vi "SLL DE Virtual Graph.vi"(8 "error in(no error)":errorcluster) -> (0 "error Out":errorcluster)   [LabVIEW 2009]
uses:
  Controls/SLL DE Get Plot LV2Global Parameters.ctl
  Sub VIs/DAQ Engine/Controls/SLL DE List of Analog Inputs.ctl
  Controls/SLL DE Virtual Graph Options.ctl
  Sub VIs/DAQ Engine/Controls/SLL DE DAQ Global Options.ctl
  Sub VIs/DAQ Engine/Controls/SLL DE DAQ Global Elements.ctl
  Controls/SLL DE Get Plot LV2Global Options.ctl
  Sub VIs/DAQ Engine/Controls/SLL DE Circular Buffer Pointers List.ctl
  Sub VIs/DAQ Engine/Controls/SLL DE Circular Buffer Options.ctl
  <vilib>/Utility/miscctls.llb/LVAnnotationListTypeDef.ctl
  Controls/SLL DE Virtual Chart Datalog Driver Options.ctl
  Sub VIs/DAQ Engine/Controls/SLL DE DO Command LV2Global Options.ctl
  Controls/SLL DE File Logging Command List.ctl
panel:
  out "Time :":string="12:11:16 PM"
  out "Date :":string="08-25-2009"
  in  "Enable Record":bool caption="Record All channels"
  in  "Plot 4":u16(ring)=19 caption="Y-Axis(1)" items=["FM01TS", "FM02TS", "FM03TS", "FM04TS", "FM05TS", "PC01TS", "PC02TS", "PC03TS", "PT01TS", "PT02TS", "PT03TS", "PT04TS", "PT05TS", "PT06TS", "ST01TS", "TC01TS", "TC02TS", "TC03TS", "TT01TS", "None"]
  in  "Plot 3":u16(ring)=19 caption="Y-Axis(1)" items=["FM01TS", "FM02TS", "FM03TS", "FM04TS", "FM05TS", "PC01TS", "PC02TS", "PC03TS", "PT01TS", "PT02TS", "PT03TS", "PT04TS", "PT05TS", "PT06TS", "ST01TS", "TC01TS", "TC02TS", "TC03TS", "TT01TS", "None"]
  in  "Plot 2":u16(ring)=19 caption="Y-Axis(1)" items=["FM01TS", "FM02TS", "FM03TS", "FM04TS", "FM05TS", "PC01TS", "PC02TS", "PC03TS", "PT01TS", "PT02TS", "PT03TS", "PT04TS", "PT05TS", "PT06TS", "ST01TS", "TC01TS", "TC02TS", "TC03TS", "TT01TS", "None"]
  in  "Y-Axis 2":bool=TRUE
  in  "Y-Axis 1":bool=TRUE
  in  "Plot 1":u16(ring) caption="Y-Axis(1)" items=["FM01TS", "FM02TS", "FM03TS", "FM04TS", "FM05TS", "PC01TS", "PC02TS", "PC03TS", "PT01TS", "PT02TS", "PT03TS", "PT04TS", "PT05TS", "PT06TS", "ST01TS", "TC01TS", "TC02TS", "TC03TS", "TT01TS", "None"]
  in  "Hold Update":bool=TRUE
  in  "X-Scale":u16(ring)=19 caption="Y-Axis(1)" items=["FM01TS", "FM02TS", "FM03TS", "FM04TS", "FM05TS", "PC01TS", "PC02TS", "PC03TS", "PT01TS", "PT02TS", "PT03TS", "PT04TS", "PT05TS", "PT06TS", "ST01TS", "TC01TS", "TC02TS", "TC03TS", "TT01TS", "Time Scale"]
  out "Graph":T1(graph)
  in  "List of Analog Inputs":T2
  in  "Data Cluster":T4={"Record"=FALSE, "Datalog Folder Path"=path "D:/Projects/Projects/Eaton Prop Valve Test Stand/Software/Info/Datalog File Path/Back up.dat", "Graph - Interval b/w Samples"=0, "AI Sampling Rate (Samples/Sec)"=3.0, "Data Log To csv File"=[], "File - Interval b/w Samples"=0, "Time Array"=[], "Graph Mod"=0, "File Mod"=0, "Plot Details"={"Sample Value In"=[], "Plot 1"=FALSE, "Plot 2"=FALSE, "Plot 3"=FALSE, "Plot 4"=FALSE}}
  in  "Data Save Folder Path":path=path "D:/STI Projects/DAQ Engine/SLL DAQ Engine/Software/Info/Report"
  in  "Snap Shot":bool caption="Duplicate SupFile"
  in  "Restart Plot":bool
  in  "Exit":bool
  in  "Print":bool
  # "Logo"
  # "Logo"
  # "<Project Name>"
  # "Graphical Display"
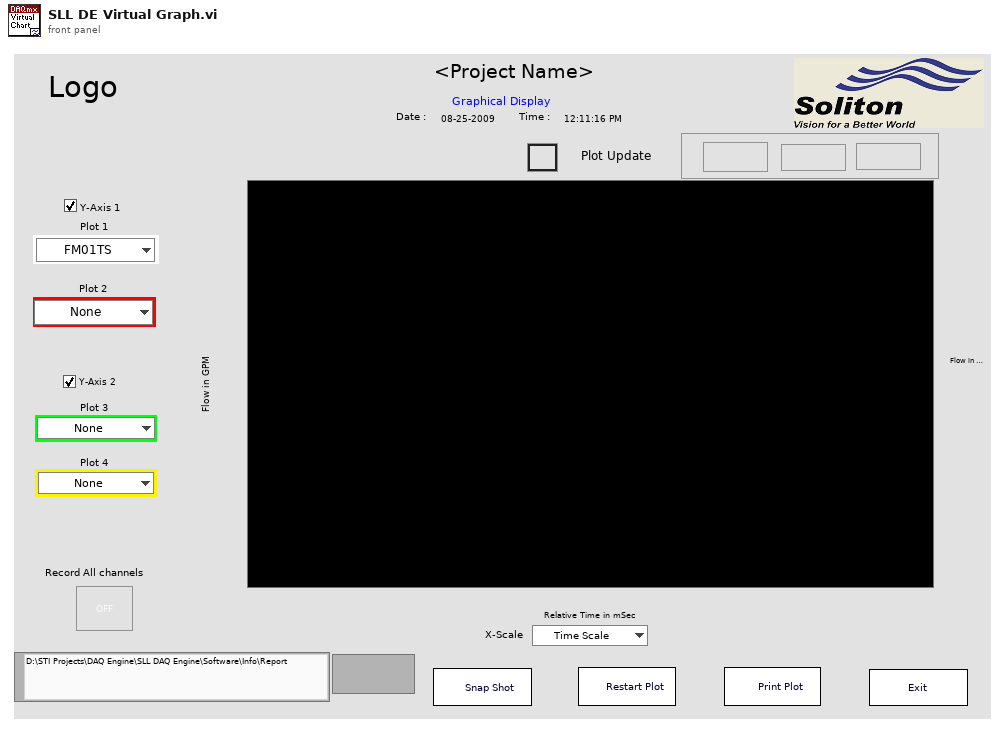
[diagram p1: front panel]
types:
  T1 = cluster{"Sample Value In":sgl[], "Sample Value In":sgl[]}[]
  T2 = typedef "SLL DE List of Analog Inputs.ctl" = enum16{"None"}
  T3 = typedef "SLL DE Get Plot LV2Global Parameters.ctl" = cluster{"Sample Value In":sgl[][], "Plot 1":bool, "Plot 2":bool, "Plot 3":bool, "Plot 4":bool}
  T4 = cluster{"Record":bool, "Datalog Folder Path":path, "Graph - Interval b/w Samples":i32, "AI Sampling Rate (Samples/Sec)":dbl, "Data Log To csv File":sgl[][], "File - Interval b/w Samples":i32, "Time Array":timestamp[], "Graph Mod":i32, "File Mod":i32, "Plot Details":T3}
  T5 = typedef "SLL DE Virtual Graph Options.ctl" = enum16{"Initialize", "Initialize Channel List", "Check Channel Type", "Update Graph Parameters", "Poll Events", "Get Values", "Config Plot", "Plot Ramp", "Datalog", "Add Plot Name", "Enable Record", "Snap Shot", "Restart", "Print Plot", "Error", "Exit"}
  T6 = typedef "SLL DE DAQ Global Options.ctl" = enum16{"Init", "Write 1", "Read 1", "Write Array", "Read Array", "Clear"}
  T7 = typedef "SLL DE DAQ Global Elements.ctl" = enum16{"AI Error", "AO Error", "DI Error", "DO Error", "AI Restart", "DI Restart", "AI Running", "AO Running", "DI Running", "DO Running", "DAQ Exit?"}
  T8 = typedef "SLL DE Get Plot LV2Global Options.ctl" = enum16{"Init", "Get Plot", "Read Plot"}
  T9 = typedef "SLL DE Circular Buffer Pointers List.ctl" = enum16{"Graph Pointer", "File Log Pointer", "Pointer 3", "Pointer 4"}
  T10 = typedef "SLL DE Circular Buffer Options.ctl" = enum16{"Initialize", "Init Pointer X", "Write", "Read Single Value", "Read Pointer X (Multi Value)", "Clear Data"}
  T11 = typedef "LVAnnotationListTypeDef.ctl" = cluster{"Name":string, "Color":u32, "Style":u8, "Point Style":u8, "Name Visible":bool, "Allow Drag":bool, "Annotation Mode":u32, "Plot":i32, "Index":i32, "Position":cluster{"X":dbl, "Y":dbl}, "X Scale":u32, "Y Scale":u32, "Show Arrow":bool, "Lock Name":bool, "Plot Area":i32, "Label Offset":cluster{"X":dbl, "Y":dbl}}[]
  T12 = typedef "SLL DE Virtual Chart Datalog Driver Options.ctl" = enum16{"Initialise", "Write Headings", "Write", "Check File Size", "Read", "Clear"}
  T13 = typedef "SLL DE File Logging Command List.ctl" = enum16{"Start Logging", "Stop Logging"}
  T14 = typedef "SLL DE DO Command LV2Global Options.ctl" = enum16{"Init/Register Events", "Get Event Refnum", "Fire Event", "Distroy Event"}
  T15 = cluster{"Plot 1":string, "Plot 2":string, "Plot 3":string, "Plot 4":string, "X Scale":string, "Y-Axis 2":bool, "Y-Axis 1":bool}
  T16 = typedef "SLL DE List of AI Channel Type.ctl" = enum16{"Pressure", "Flow", "Temperature", "Time Scale", "Voltage", "Current", "Frequency", "Sound", "Speed", "Torque", "Distance", "Channel Type 1", "Channel Type 2", "Channel Type 3"}
  T17 = cluster{"Time Scale":sgl[], "Sample Value In":sgl[]}[]
  T18 = enum16{"Left Button", "Center Button", "Right Button", "Window Close"}
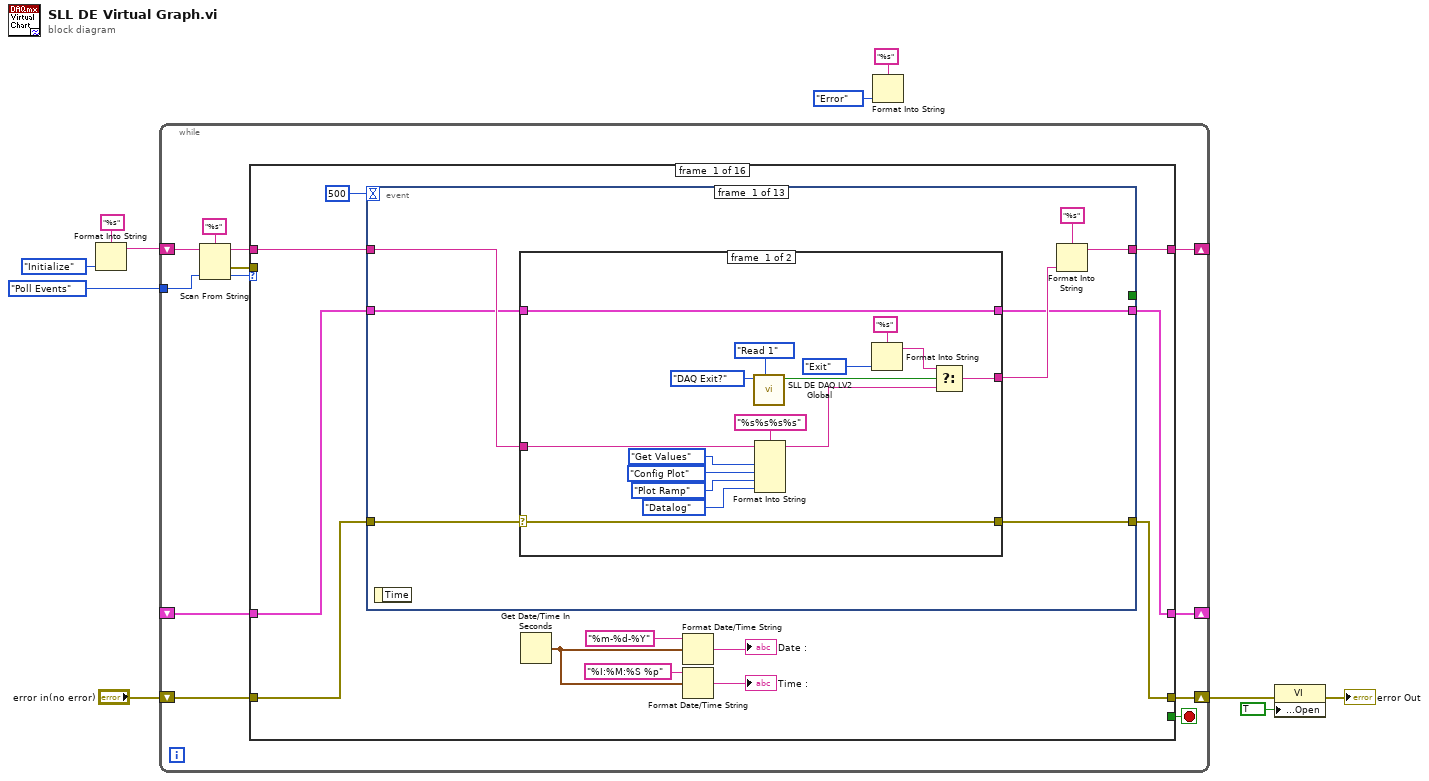
[diagram p0: block diagram]
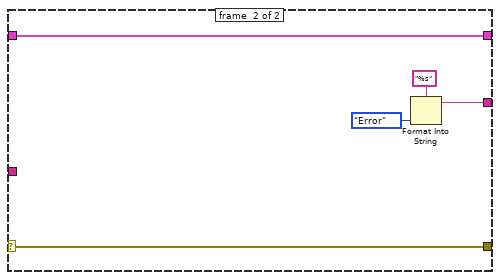
[diagram p2: hidden frame]
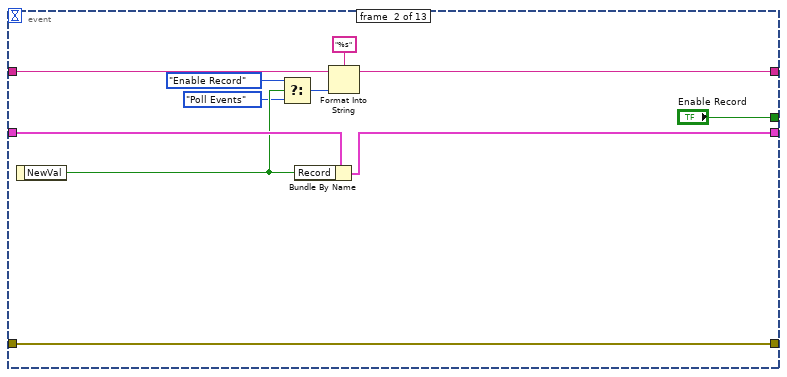
[diagram p3: hidden frame]
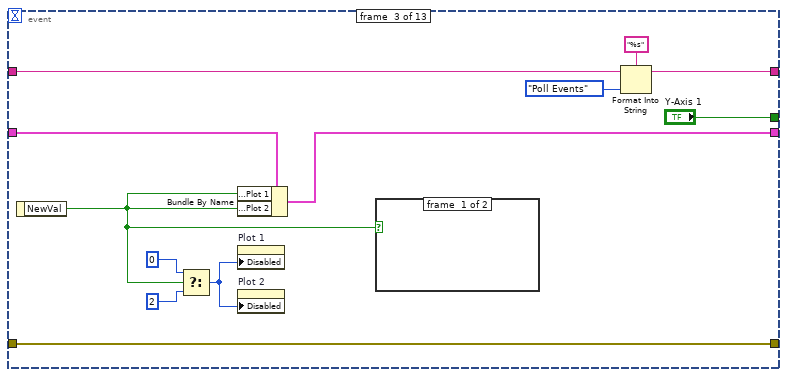
[diagram p4: hidden frame]
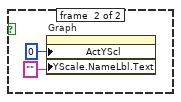
[diagram p5: hidden frame]
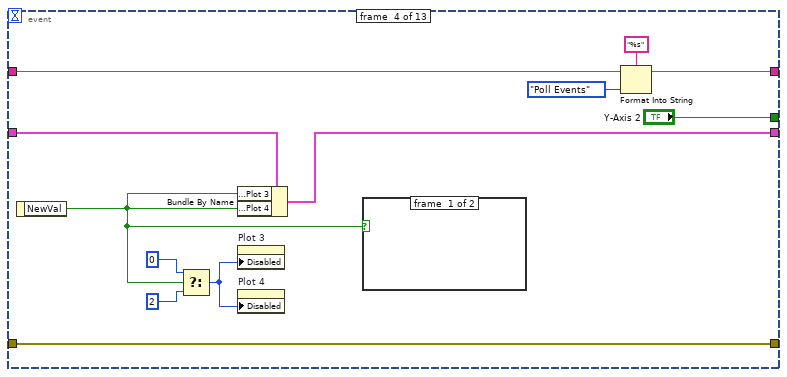
[diagram p6: hidden frame]
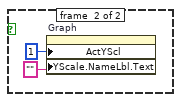
[diagram p7: hidden frame]
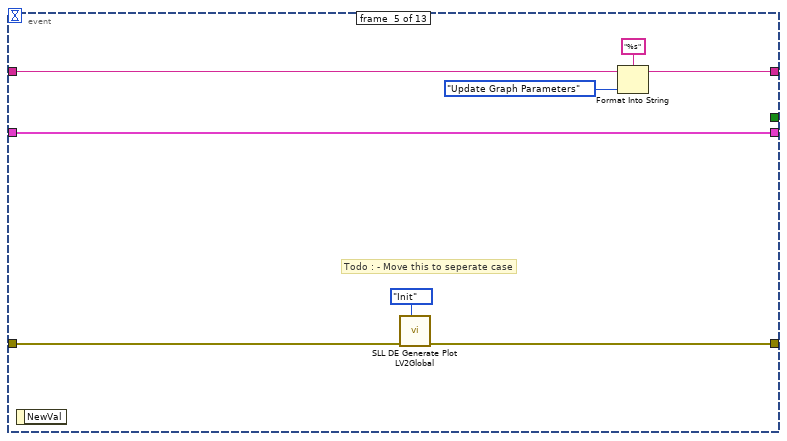
[diagram p8: hidden frame]
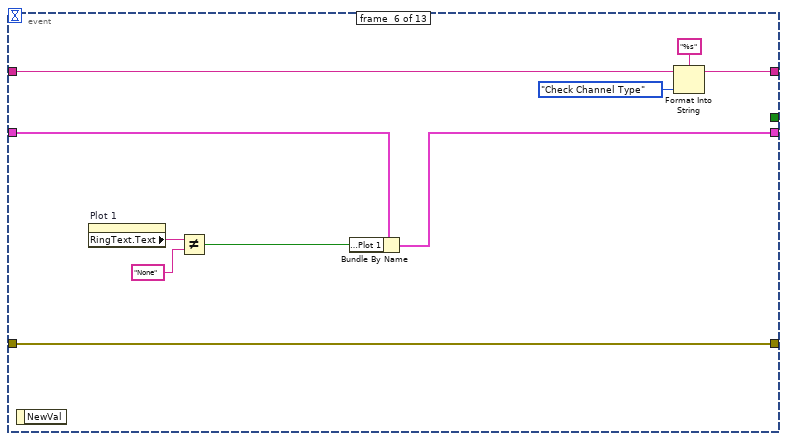
[diagram p9: hidden frame]
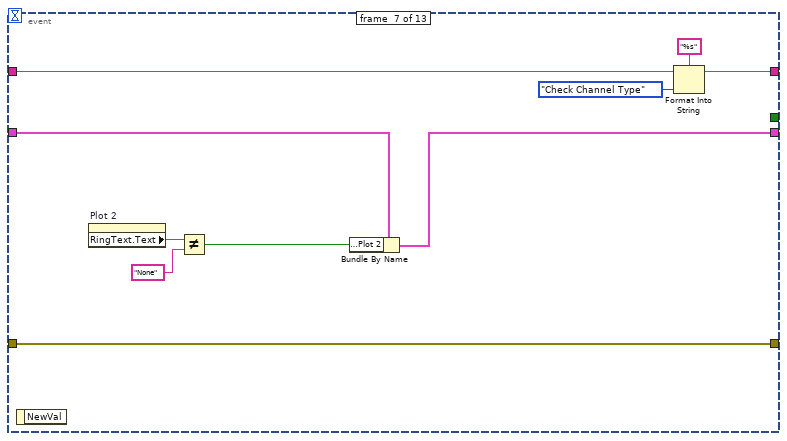
[diagram p10: hidden frame]
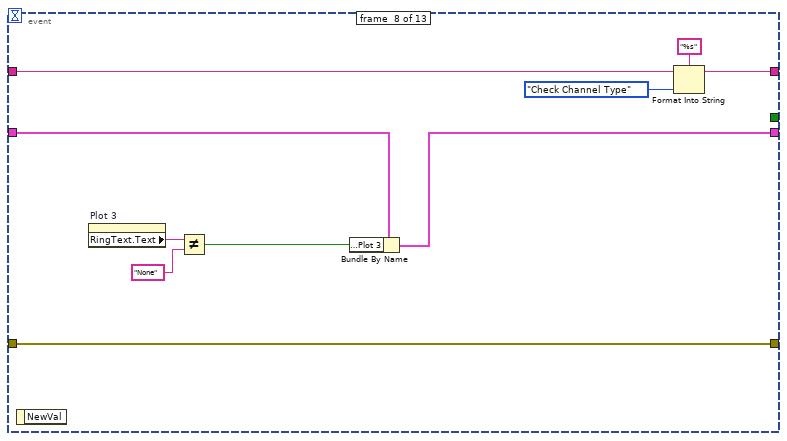
[diagram p11: hidden frame]
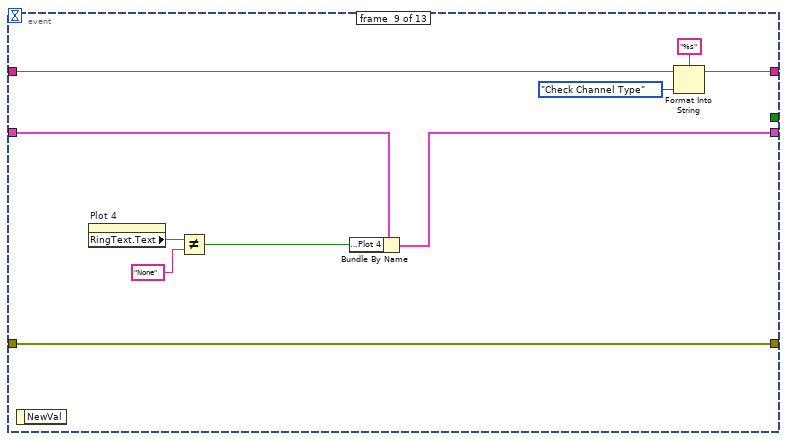
[diagram p12: hidden frame]
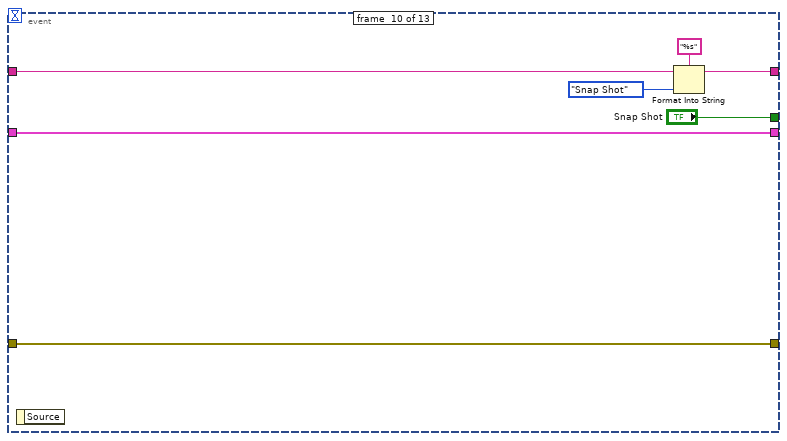
[diagram p13: hidden frame]
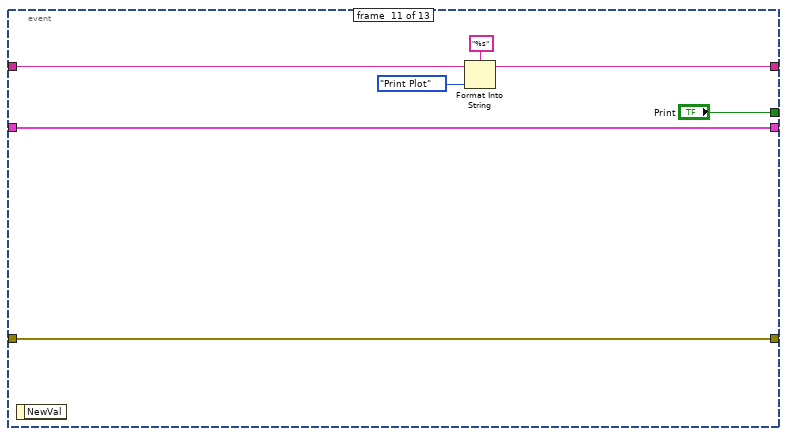
[diagram p14: hidden frame]
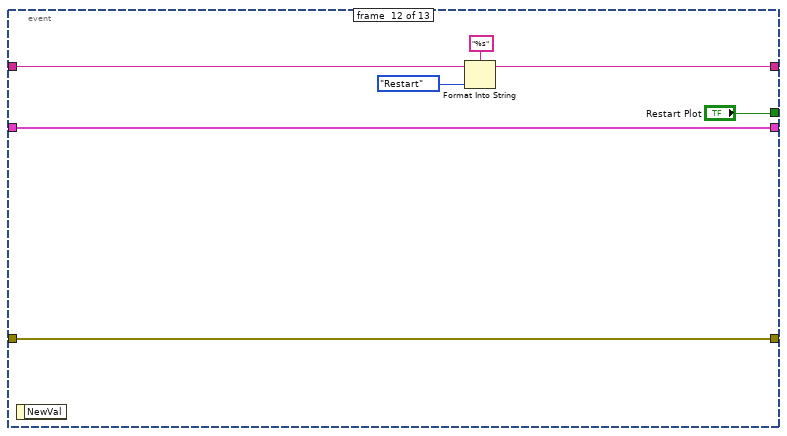
[diagram p15: hidden frame]
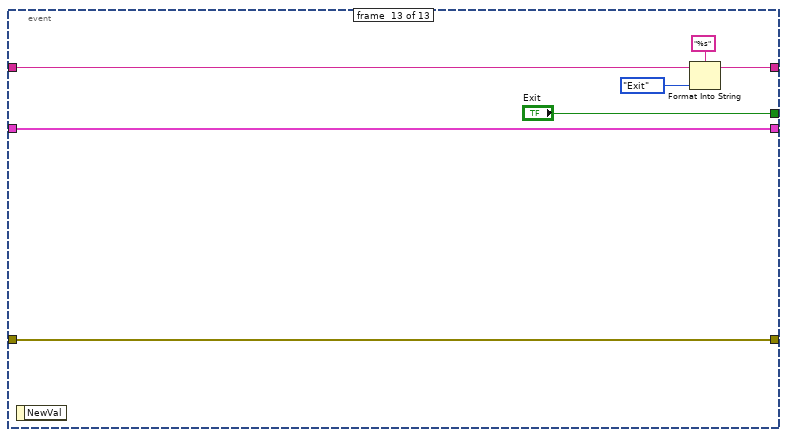
[diagram p16: hidden frame]
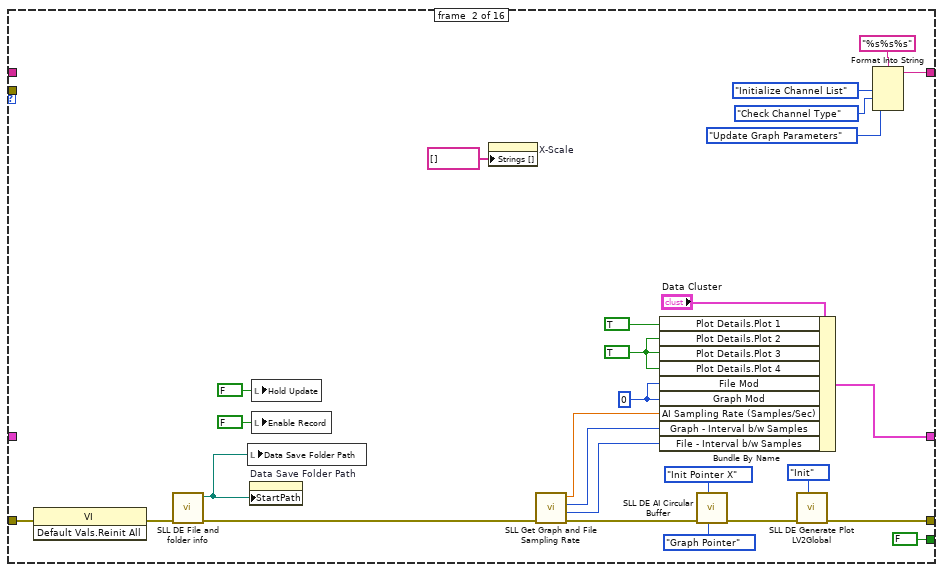
[diagram p17: hidden frame]
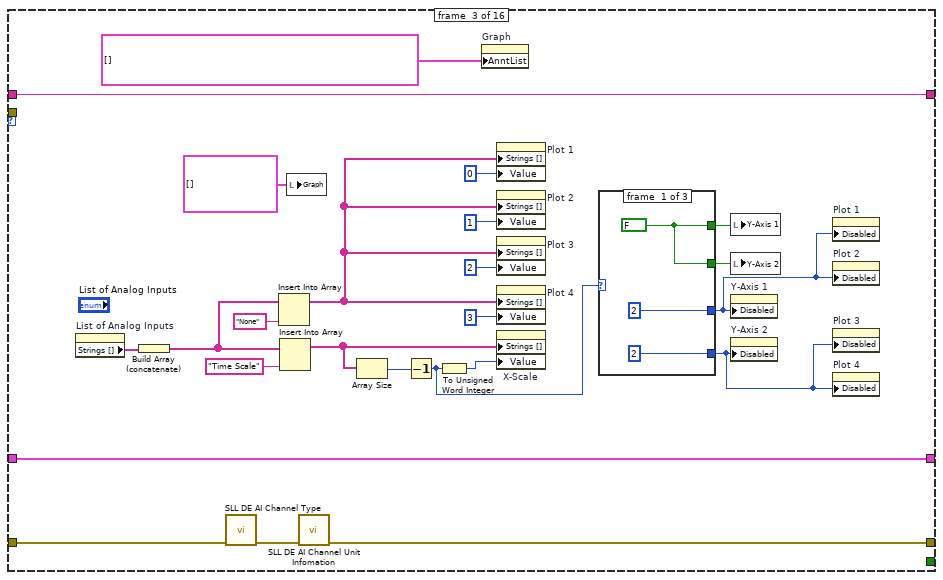
[diagram p18: hidden frame]
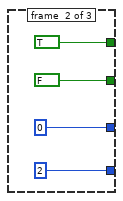
[diagram p19: hidden frame]
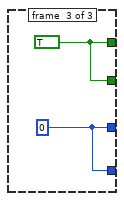
[diagram p20: hidden frame]
diagram:
  n1 = Format Into String(format string="%s", SLL_DE_Virtual_Graph_Options."Initialize" ("SLL DE Virtual Chart Options")) -> (resulting string=w10:string)  [unwired: 2 in, 1 out]
  n2 = while {
    shift-right: [w19] -> _
    shift-left: w10 -> [w22]
    shift-right: [w18] -> _
    shift-left: _ -> [w16]
    shift-right: [w15] -> w8
    shift-left: "error in(no error)" -> [w14]
    tunnel: SLL_DE_Virtual_Graph_Options."Poll Events" ("SLL DE Virtual Chart Options") -> [w12]
    stop <- w17 stop-if-true
    n3 = Scan From String(format string="%s", input string=w22, default 1=w12) -> (remaining string=w20:string, error out=w13:errorcluster, output 1=w21:T5)  [unwired: 2 in, 1 out]
    n4 = case shown="\"Initialize\"" w21 {
      tunnel: w20 -> [w33 _ w217 w257 _ w349 w379 w391 w414 w428 w450 w464 _ w495 _ w513]
      tunnel: [w32 w198 w217 w256 w292 w349 w379 w391 w414 w428 w450 w464 w465 w495 w497 w513] -> w19
      tunnel: [w30 w202 w216 w249 w300 w350 w380 w387 w413 w425 w449 w461 w478 w484 w498 w512] -> w18
      tunnel: [_ FALSE _ _ _ _ _ _ _ _ _ _ FALSE _ _ TRUE] -> w17
      tunnel: w16 -> [w31 _ w216 w250 w300 w344 w381 w387 w413 w425 w449 w461 w478 w484 w498 w512]
      tunnel: [w28 w192 w209 w261 w299 w345 w375 w386 w418 w426 w440 w451 w474 w480 w496 w508] -> w15
      tunnel: w14 -> [w29 w205 w211 w261 w301 w346 w378 w390 w419 w427 w434 w454 w475 w485 w500 w509]
      tunnel: w13 -> [_ _ _ _ _ _ _ _ _ _ _ _ _ _ _ _]
      frame #0 {
        n5 = event shown="[5] \"Plot 1\": Value Change" {
          selector: _ -> [_ _ _ _ _ _ _ _ _ _ _ _ _]
          dyn-events: _ -> [_ _ _ _ _ _ _ _ _ _ _ _ _]
          timeout: 500 -> [_ _ _ _ _ _ _ _ _ _ _ _ _]
          tunnel: w33 -> [w39 w64 w81 w91 w107 w111 w121 w131 w141 w153 w158 w166 w172]
          tunnel: [w41 w73 w82 w92 w109 w119 w122 w132 w142 w154 w162 w170 w177] -> w32
          tunnel: [_ "Enable Record" "Y-Axis 1" "Y-Axis 2" _ _ _ _ _ "Snap Shot" "Print" "Restart Plot" "Exit"] -> _
          tunnel: w31 -> [w37 w71 w85 w90 w103 w118 w125 w135 w145 w152 w161 w169 w175]
          tunnel: [w36 w70 w84 w93 w103 w117 w123 w133 w143 w152 w161 w169 w175] -> w30
          tunnel: w29 -> [w38 w69 w79 w94 w105 w116 w124 w134 w144 w155 w160 w168 w174]
          tunnel: [w35 w69 w79 w94 w104 w116 w124 w134 w144 w155 w160 w168 w174] -> w28
          event #0 {
            n6 = event-data() -> ()  [unwired: 1 in, 1 out]
            n7 = case shown="No Error" w38 {
              selector: w38 -> [w43 w59]
              tunnel: [w58 w61] -> w40
              tunnel: w39 -> [w45 _]
              tunnel: w37 -> [w44 w60]
              tunnel: [w44 w60] -> w36
              tunnel: [w43 w59] -> w35
              frame #0 {
                n8 = call "SLL DE DAQ LV2 Global.vi"("Option"=SLL_DE_DAQ_Global_Options."Read 1", "Element"=SLL_DE_DAQ_Global_Elements."DAQ Exit?") -> ("Status Out"=w55:bool)  [unwired: 7 in, 2 out]
                n9 = Format Into String(format string="%s%s%s%s", initial string=w45, SLL_DE_Virtual_Graph_Options."Get Values" ("SLL DE Virtual Chart Options"), SLL_DE_Virtual_Graph_Options."Config Plot" ("SLL DE Virtual Chart Options"), SLL_DE_Virtual_Graph_Options."Plot Ramp" ("SLL DE Virtual Chart Options"), SLL_DE_Virtual_Graph_Options."Datalog" ("SLL DE Virtual Chart Options")) -> (resulting string=w49:string)  [unwired: 1 in, 1 out]
                n10 = Format Into String(format string="%s", SLL_DE_Virtual_Graph_Options."Exit" ("SLL DE Virtual Chart Options")) -> (resulting string=w46:string)  [unwired: 2 in, 1 out]
                n11 = Select(t=w46, s=w55, f=w49) -> (s? t:f=w58:string)
              }
              frame #1 {
                n12 = Format Into String(format string="%s", SLL_DE_Virtual_Graph_Options."Error" ("SLL DE Virtual Chart Options")) -> (resulting string=w61:string)  [unwired: 2 in, 1 out]
              }
            }
            n13 = Format Into String(format string="%s", w40) -> (resulting string=w41:string)  [unwired: 2 in, 1 out]
          }
          event #1 {
            n14 = event-data() -> ("NewVal"=w67:bool)  [unwired: 1 in]
            n15 = Select(t=SLL_DE_Virtual_Graph_Options."Enable Record" ("SLL DE Virtual Chart Options"), s=w67, f=SLL_DE_Virtual_Graph_Options."Poll Events") -> (s? t:f=w66:T5)
            n16 = Bundle By Name(cluster=w71, "Record"=w67) -> (w70:T4)
            n17 = Format Into String(format string="%s", initial string=w64, w66) -> (resulting string=w73:string)  [unwired: 1 in, 1 out]
          }
          event #2 {
            n18 = event-data() -> ("NewVal"=w75:bool)  [unwired: 1 in]
            n19 = Select(t=u8 0 ("Disabled"), s=w75, f=u8 2 ("Disabled")) -> (s? t:f=w77:u8)
            n20 = Bundle By Name(cluster=w85, "Plot Details.Plot 1"=w75, "Plot Details.Plot 2"=w75) -> (w84:T4)
            n21 = property on="Plot 1" class="Ring (strict)"("Disabled"=w77) -> ()  [unwired: 2 in, 2 out]
            n22 = property on="Plot 2" class="Ring (strict)"("Disabled"=w77) -> ()  [unwired: 2 in, 2 out]
            n23 = case shown="True" w75 {
              frame #0 {
              }
              frame #1 {
                n24 = property on="Graph" class="XYGraph (strict)"("ActYScl"=0 ("Active Y Scale"), "YScale.NameLbl.Text"="" ("Y Scale.Name Label.Text")) -> ()  [unwired: 2 in, 2 out]
              }
            }
            n25 = Format Into String(format string="%s", initial string=w81, SLL_DE_Virtual_Graph_Options."Poll Events" ("SLL DE Virtual Chart Options")) -> (resulting string=w82:string)  [unwired: 1 in, 1 out]
          }
          event #3 {
            n26 = event-data() -> ("NewVal"=w89:bool)  [unwired: 1 in]
            n27 = Select(t=u8 0 ("Disabled"), s=w89, f=u8 2 ("Disabled")) -> (s? t:f=w96:u8)
            n28 = Bundle By Name(cluster=w90, "Plot Details.Plot 3"=w89, "Plot Details.Plot 4"=w89) -> (w93:T4)
            n29 = property on="Plot 3" class="Ring (strict)"("Disabled"=w96) -> ()  [unwired: 2 in, 2 out]
            n30 = property on="Plot 4" class="Ring (strict)"("Disabled"=w96) -> ()  [unwired: 2 in, 2 out]
            n31 = case shown="True" w89 {
              frame #0 {
              }
              frame #1 {
                n32 = property on="Graph" class="XYGraph (strict)"("ActYScl"=1 ("Active Y Scale"), "YScale.NameLbl.Text"="" ("Y Scale.Name Label.Text")) -> ()  [unwired: 2 in, 2 out]
              }
            }
            n33 = Format Into String(format string="%s", initial string=w91, SLL_DE_Virtual_Graph_Options."Poll Events" ("SLL DE Virtual Chart Options")) -> (resulting string=w92:string)  [unwired: 1 in, 1 out]
          }
          event #4 {
            # "Todo : - Move this to seperate case"
            n34 = event-data() -> ()  [unwired: 1 in, 1 out]
            n35 = call "SLL DE Generate Plot LV2Global.vi"("Option"=SLL_DE_Get_Plot_LV2Global_Options."Init", "error in (no error)"=w105) -> ("error IO"=w104:errorcluster)  [unwired: 8 in, 1 out]
            n36 = Format Into String(format string="%s", initial string=w107, SLL_DE_Virtual_Graph_Options."Update Graph Parameters" ("SLL DE Virtual Chart Options")) -> (resulting string=w109:string)  [unwired: 1 in, 1 out]
          }
          event #5 {
            n37 = event-data() -> ()  [unwired: 1 in, 1 out]
            n38 = property on="Plot 1" class="Ring (strict)"() -> ("RingText.Text"=w115:string)  [unwired: 2 in, 2 out]
            n39 = Not Equal?(x=w115, y="None") -> (x != y?=w113:bool)
            n40 = Bundle By Name(cluster=w118, "Plot Details.Plot 1"=w113) -> (w117:T4)
            n41 = Format Into String(format string="%s", initial string=w111, SLL_DE_Virtual_Graph_Options."Check Channel Type" ("SLL DE Virtual Chart Options")) -> (resulting string=w119:string)  [unwired: 1 in, 1 out]
          }
          event #6 {
            n42 = event-data() -> ()  [unwired: 1 in, 1 out]
            n43 = property on="Plot 2" class="Ring (strict)"() -> ("RingText.Text"=w129:string)  [unwired: 2 in, 2 out]
            n44 = Not Equal?(x=w129, y="None") -> (x != y?=w127:bool)
            n45 = Bundle By Name(cluster=w125, "Plot Details.Plot 2"=w127) -> (w123:T4)
            n46 = Format Into String(format string="%s", initial string=w121, SLL_DE_Virtual_Graph_Options."Check Channel Type" ("SLL DE Virtual Chart Options")) -> (resulting string=w122:string)  [unwired: 1 in, 1 out]
          }
          event #7 {
            n47 = event-data() -> ()  [unwired: 1 in, 1 out]
            n48 = property on="Plot 3" class="Ring (strict)"() -> ("RingText.Text"=w139:string)  [unwired: 2 in, 2 out]
            n49 = Not Equal?(x=w139, y="None") -> (x != y?=w137:bool)
            n50 = Bundle By Name(cluster=w135, "Plot Details.Plot 3"=w137) -> (w133:T4)
            n51 = Format Into String(format string="%s", initial string=w131, SLL_DE_Virtual_Graph_Options."Check Channel Type" ("SLL DE Virtual Chart Options")) -> (resulting string=w132:string)  [unwired: 1 in, 1 out]
          }
          event #8 {
            n52 = event-data() -> ()  [unwired: 1 in, 1 out]
            n53 = property on="Plot 4" class="Ring (strict)"() -> ("RingText.Text"=w149:string)  [unwired: 2 in, 2 out]
            n54 = Not Equal?(x=w149, y="None") -> (x != y?=w147:bool)
            n55 = Bundle By Name(cluster=w145, "Plot Details.Plot 4"=w147) -> (w143:T4)
            n56 = Format Into String(format string="%s", initial string=w141, SLL_DE_Virtual_Graph_Options."Check Channel Type" ("SLL DE Virtual Chart Options")) -> (resulting string=w142:string)  [unwired: 1 in, 1 out]
          }
          event #9 {
            n57 = event-data() -> ()  [unwired: 1 in, 1 out]
            n58 = Format Into String(format string="%s", initial string=w153, SLL_DE_Virtual_Graph_Options."Snap Shot" ("SLL DE Virtual Chart Options")) -> (resulting string=w154:string)  [unwired: 1 in, 1 out]
          }
          event #10 {
            n59 = event-data() -> ()  [unwired: 1 in, 1 out]
            n60 = Format Into String(format string="%s", initial string=w158, SLL_DE_Virtual_Graph_Options."Print Plot" ("SLL DE Virtual Chart Options")) -> (resulting string=w162:string)  [unwired: 1 in, 1 out]
          }
          event #11 {
            n61 = event-data() -> ()  [unwired: 1 in, 1 out]
            n62 = Format Into String(format string="%s", initial string=w166, SLL_DE_Virtual_Graph_Options."Restart" ("SLL DE Virtual Chart Options")) -> (resulting string=w170:string)  [unwired: 1 in, 1 out]
          }
          event #12 {
            n63 = event-data() -> ()  [unwired: 1 in, 1 out]
            n64 = Format Into String(format string="%s", initial string=w172, SLL_DE_Virtual_Graph_Options."Exit" ("SLL DE Virtual Chart Options")) -> (resulting string=w177:string)  [unwired: 1 in, 1 out]
          }
        }
        n65 = Get Date/Time In Seconds() -> (seconds since 1Jan1904=w25:timestamp)
        n66 = Format Date/Time String(time format string (%c)="%m-%d-%Y", seconds (now)=w25) -> (date/time string=→"Date :":string)  [unwired: 1 in]
        n67 = Format Date/Time String(time format string (%c)="%I:%M:%S %p", seconds (now)=w25) -> (date/time string=→"Time :":string)  [unwired: 1 in]
      }
      frame #1 {
        w190 = TRUE ("Data Cluster 2.Plot 1")
        w195 = 0 ("Mod")
        n68 = invoke class="VI" method="Default Vals.Reinit All"(error in=w205) -> (error out=w204:errorcluster)  [unwired: 2 in, 2 out]
        n69 = call "SLL DE File and folder info.vi"("error in (no error)"=w204) -> ("error out"=w187:errorcluster, "Report path"=w181:path)  [unwired: 5 in, 4 out]
        n70 = local write "Data Save Folder Path"(w181) -> ()
        n71 = property on="Data Save Folder Path" class="Path"("StartPath"=w181) -> ()  [unwired: 2 in, 2 out]
        n72 = local write "Hold Update"(FALSE ("Hold Update")) -> ()
        n73 = local write "Enable Record"(FALSE ("Enable Record")) -> ()
        n74 = property on="X-Scale" class="Ring (strict)"("Strings []"=string[] []) -> ()  [unwired: 2 in, 2 out]
        n75 = call "SLL Get Graph and File Sampling Rate.vi"("error in (no error)"=w187) -> ("error out"=w186:errorcluster, "File - Interval b/w Samples"=w184:i32, "Graph - Interval b/w Samples"=w179:i32, "AI Sampling Rate (Samples/Sec)"=w185:dbl)  [unwired: 7 in]
        n76 = Bundle By Name(cluster="Data Cluster", "Plot Details.Plot 1"=TRUE ("Data Cluster 2.Plot 1"), "Plot Details.Plot 2"=w190, "Plot Details.Plot 3"=w190, "Plot Details.Plot 4"=w190, "File Mod"=w195, "Graph Mod"=w195, "AI Sampling Rate (Samples/Sec)"=w185, "Graph - Interval b/w Samples"=w179, "File - Interval b/w Samples"=w184) -> (w202:T4)
        n77 = call "SLL DE AI Circular Buffer.vi"("Pointers"=SLL_DE_Circular_Buffer_Pointers_List."Graph Pointer", "Options"=SLL_DE_Circular_Buffer_Options."Init Pointer X" ("AI Option"), "error in (no error)"=w186) -> ("error Out"=w193:errorcluster)  [unwired: 3 in, 5 out]
        n78 = call "SLL DE Generate Plot LV2Global.vi"("Option"=SLL_DE_Get_Plot_LV2Global_Options."Init", "error in (no error)"=w193) -> ("error IO"=w192:errorcluster)  [unwired: 8 in, 1 out]
        n79 = Format Into String(format string="%s%s%s", SLL_DE_Virtual_Graph_Options."Initialize Channel List" ("SLL DE Virtual Chart Options"), SLL_DE_Virtual_Graph_Options."Check Channel Type" ("SLL DE Virtual Chart Options"), SLL_DE_Virtual_Graph_Options."Update Graph Parameters" ("SLL DE Virtual Chart Options")) -> (resulting string=w198:string)  [unwired: 2 in, 1 out]
      }
      frame #2 {
        n80 = property on="List of Analog Inputs" class="Enum (strict)"() -> ("Strings []"=w221:string[])  [unwired: 2 in, 2 out]
        n81 = Build Array (concatenate)(w221) -> (w220:string[])
        n82 = call "SLL DE AI Channel Type.vi"("error in (no error)"=w211) -> ("error out"=w210:errorcluster)  [unwired: 7 in, 3 out]
        n83 = Insert Into Array(array=w220, new element="None") -> (w222:string[])  [unwired: 1 in]
        n84 = Insert Into Array(array=w220, new element="Time Scale") -> (w223:string[])  [unwired: 1 in]
        n85 = local write "Graph"(T1 [] ("Graph")) -> ()
        n86 = call "SLL DE AI Channel Unit Infomation.vi"("error in (no error)"=w210) -> ("error out"=w209:errorcluster)  [unwired: 9 in, 1 out]
        n87 = Array Size(array=w223) -> (size(s)=w224:i32)
        n88 = Decrement(x=w224) -> (x-1=w226:i32)
        n89 = To Unsigned Word Integer(number=w226) -> (unsigned 16bit integer=w225:u16)
        n90 = property on="Graph" class="XYGraph (strict)"("AnntList"=T11 [] ("Annotation List")) -> ()  [unwired: 2 in, 2 out]
        n91 = property on="Plot 1" class="Ring (strict)"("Strings []"=w222, "Value"=u16 0) -> ()  [unwired: 2 in, 2 out]
        n92 = property on="Plot 2" class="Ring (strict)"("Strings []"=w222, "Value"=u16 1) -> ()  [unwired: 2 in, 2 out]
        n93 = property on="Plot 3" class="Ring (strict)"("Strings []"=w222, "Value"=u16 2) -> ()  [unwired: 2 in, 2 out]
        n94 = property on="Plot 4" class="Ring (strict)"("Strings []"=w222, "Value"=u16 3) -> ()  [unwired: 2 in, 2 out]
        n95 = property on="X-Scale" class="Ring (strict)"("Strings []"=w223, "Value"=w225) -> ()  [unwired: 2 in, 2 out]
        n96 = case shown="0" w226 {
          tunnel: [w232 TRUE w238] -> w227
          tunnel: [w232 FALSE w238] -> w228
          tunnel: [u8 2 ("Disabled") u8 0 ("Disabled") w237] -> w208
          tunnel: [u8 2 ("Disabled") u8 2 ("Disabled") w237] -> w207
          frame #0 {
            w232 = FALSE
          }
          frame #1 {
          }
          frame #2 {
            w237 = u8 0 ("Disabled")
            w238 = TRUE
          }
        }
        n97 = local write "Y-Axis 1"(w227) -> ()
        n98 = local write "Y-Axis 2"(w228) -> ()
        n99 = property on="Y-Axis 1" class="Bool (strict)"("Disabled"=w208) -> ()  [unwired: 2 in, 2 out]
        n100 = property on="Y-Axis 2" class="Bool (strict)"("Disabled"=w207) -> ()  [unwired: 2 in, 2 out]
        n101 = property on="Plot 1" class="Ring (strict)"("Disabled"=w208) -> ()  [unwired: 2 in, 2 out]
        n102 = property on="Plot 2" class="Ring (strict)"("Disabled"=w208) -> ()  [unwired: 2 in, 2 out]
        n103 = property on="Plot 3" class="Ring (strict)"("Disabled"=w207) -> ()  [unwired: 2 in, 2 out]
        n104 = property on="Plot 4" class="Ring (strict)"("Disabled"=w207) -> ()  [unwired: 2 in, 2 out]
      }
      frame #3 {
        n105 = Unbundle By Name(w250) -> ("Plot Details.Plot 2"=w252:bool, "Plot Details.Plot 4"=w251:bool)
        n106 = property on="Plot 3" class="Ring (strict)"() -> ("RingText.Text"=w254:string)  [unwired: 2 in, 2 out]
        n107 = property on="Plot 4" class="Ring (strict)"() -> ("RingText.Text"=w253:string)  [unwired: 2 in, 2 out]
        n108 = property on="Plot 1" class="Ring (strict)"() -> ("RingText.Text"=w255:string)  [unwired: 2 in, 2 out]
        n109 = property on="Plot 2" class="Ring (strict)"() -> ("RingText.Text"=w260:string)  [unwired: 2 in, 2 out]
        n110 = case shown="Default" w254 {
          selector: w254 -> [_ w267]
          tunnel: w253 -> [_ w271]
          tunnel: [FALSE TRUE] -> w242
          tunnel: [w262 w265] -> w241
          tunnel: w251 -> [w262 w264]
          frame #0 {
          }
          frame #1 {
            n111 = call "SLL DE Virtual Graph Channel Parameters.vi"("Virtual Channel Name"=w267) -> ("Channel Type"=w270:T16)  [unwired: 5 in, 5 out]
            n112 = call "SLL DE Virtual Graph Channel Parameters.vi"("Virtual Channel Name"=w271) -> ("Channel Type"=w269:T16)  [unwired: 5 in, 5 out]
            n113 = Not Equal?(x=w270, y=w269) -> (x != y?=w268:bool)
            n114 = case shown="True" w268 {
              tunnel: [w272 FALSE] -> w265
              tunnel: w264 -> [w272 _]
              frame #0 {
              }
              frame #1 {
                n115 = property on="Plot 2" class="Ring (strict)"() -> ("NumItems"=w274:u32)  [unwired: 2 in, 2 out]
                n116 = Decrement(x=w274) -> (x-1=w273:u32)
                n117 = local write "Plot 4"(w273) -> ()
              }
            }
          }
        }
        n118 = case shown="Default" w255 {
          selector: w255 -> [_ w281]
          tunnel: w260 -> [_ w285]
          tunnel: [FALSE TRUE] -> w247
          tunnel: [w276 w279] -> w246
          tunnel: w252 -> [w276 w278]
          frame #0 {
          }
          frame #1 {
            n119 = call "SLL DE Virtual Graph Channel Parameters.vi"("Virtual Channel Name"=w281) -> ("Channel Type"=w284:T16)  [unwired: 5 in, 5 out]
            n120 = call "SLL DE Virtual Graph Channel Parameters.vi"("Virtual Channel Name"=w285) -> ("Channel Type"=w283:T16)  [unwired: 5 in, 5 out]
            n121 = Not Equal?(x=w284, y=w283) -> (x != y?=w282:bool)
            n122 = case shown="True" w282 {
              tunnel: [w286 FALSE] -> w279
              tunnel: w278 -> [w286 _]
              frame #0 {
              }
              frame #1 {
                n123 = property on="Plot 2" class="Ring (strict)"() -> ("NumItems"=w288:u32)  [unwired: 2 in, 2 out]
                n124 = Decrement(x=w288) -> (x-1=w287:u32)
                n125 = local write "Plot 2"(w287) -> ()
              }
            }
          }
        }
        n126 = local read "Y-Axis 1"() -> (w245:bool)
        n127 = local read "Y-Axis 2"() -> (w240:bool)
        n128 = And(x=w245, y=w247) -> (x .and. y?=w248:bool)
        n129 = And(x=w245, y=w246) -> (x .and. y?=w244:bool)
        n130 = And(x=w242, y=w240) -> (x .and. y?=w243:bool)
        n131 = And(x=w240, y=w241) -> (x .and. y?=w239:bool)
        n132 = Bundle By Name(cluster=w250, "Plot Details.Plot 1"=w248, "Plot Details.Plot 2"=w244, "Plot Details.Plot 3"=w243, "Plot Details.Plot 4"=w239) -> (w249:T4)
        n133 = Format Into String(format string="%s", initial string=w257, SLL_DE_Virtual_Graph_Options."Update Graph Parameters" ("SLL DE Virtual Chart Options")) -> (resulting string=w256:string)  [unwired: 1 in, 1 out]
      }
      frame #4 {
        n134 = property on="X-Scale" class="Ring (strict)"(error in=w301) -> (error out=w298:errorcluster, "RingText.Text"=w291:string)  [unwired: 1 in, 1 out]
        n135 = property on="Plot 1" class="Ring (strict)"(error in=w301) -> (error out=w302:errorcluster, "RingText.Text"=w303:string)  [unwired: 1 in, 1 out]
        n136 = property on="Plot 3" class="Ring (strict)"(error in=w301) -> ("RingText.Text"=w304:string)  [unwired: 1 in, 2 out]
        n137 = Build Array(w303, w304) -> (w305:string[])
        n138 = case shown="Default" w291 {
          selector: w291 -> [_ w308]
          tunnel: w298 -> [w307 w310]
          frame #0 {
            n139 = property on="Graph" class="XYGraph (strict)"(error in=w307, "XScale.NameLbl.Text"="Relative Time in mSec" ("X Scale.Name Label.Text")) -> ()  [unwired: 1 in, 2 out]
          }
          frame #1 {
            n140 = call "SLL DE Virtual Graph Channel Parameters.vi"("error in (no error)"=w310, "Virtual Channel Name"=w308) -> ("error out"=w309:errorcluster, "Maximum Value"=w312:dbl, "Minimum Value"=w313:dbl, "Graph Name Label"=w314:string, "Increment"=w311:dbl)  [unwired: 4 in, 1 out]
            n141 = property on="Graph" class="XYGraph (strict)"(error in=w309, "XScale.NameLbl.Text"=w314, "XScale.Minimum"=w313, "XScale.Maximum"=w312, "XScale.Increment"=w311) -> ()  [unwired: 1 in, 2 out]
          }
        }
        n142 = for {
          tunnel: w305 -> [w319] mode=indexing
          shift-right: [w318] -> w299
          shift-left: w302 -> [w317]
          i -> [w320]
          n143 = property on="Graph" class="XYGraph (strict)"(error in=w317, "ActYScl"=w320) -> (error out=w316:errorcluster)  [unwired: 1 in, 1 out]
          n144 = call "SLL DE Virtual Graph Channel Parameters.vi"("error in (no error)"=w316, "Virtual Channel Name"=w319) -> ("error out"=w315:errorcluster, "Maximum Value"=w323:dbl, "Minimum Value"=w322:dbl, "Graph Name Label"=w321:string, "Increment"=w324:dbl)  [unwired: 4 in, 1 out]
          n145 = property on="Graph" class="XYGraph (strict)"(error in=w315, "YScale.NameLbl.Text"=w321, "YScale.Minimum"=w322, "YScale.Maximum"=w323, "YScale.Increment"=w324) -> (error out=w318:errorcluster)  [unwired: 1 in, 1 out]
        }
        n146 = Format Into String(format string="%s%s%s%s%s", SLL_DE_Virtual_Graph_Options."Get Values" ("SLL DE Virtual Chart Options"), SLL_DE_Virtual_Graph_Options."Config Plot" ("SLL DE Virtual Chart Options"), SLL_DE_Virtual_Graph_Options."Plot Ramp" ("SLL DE Virtual Chart Options"), SLL_DE_Virtual_Graph_Options."Datalog" ("SLL DE Virtual Chart Options"), SLL_DE_Virtual_Graph_Options."Add Plot Name" ("SLL DE Virtual Chart Options")) -> (resulting string=w292:string)  [unwired: 2 in, 1 out]
      }
      frame #5 {
        n147 = call "SLL DE AI Circular Buffer.vi"("Pointers"=SLL_DE_Circular_Buffer_Pointers_List."Graph Pointer", "Options"=SLL_DE_Circular_Buffer_Options."Read Pointer X (Multi Value)" ("AI Option"), "error in (no error)"=w346) -> ("error Out"=w345:errorcluster, "Output Data"=w343:sgl[][], "Multi Time Stamp"=w330:timestamp[])  [unwired: 3 in, 3 out]
        n148 = Unbundle By Name(w344) -> ("Graph Mod"=w337:i32, "Graph - Interval b/w Samples"=w340:i32, "Record"=w336:bool, "File Mod"=w335:i32, "File - Interval b/w Samples"=w333:i32)
        n149 = Transpose 2D Array(2D array=w343) -> (transposed array=w329:sgl[][])
        n150 = Array Size(array=w329) -> (size(s)=w342:i32[])
        n151 = Index Array(array=w342) -> (element #1=w331:i32, element #2=w332:i32)  [unwired: 2 in]
        n152 = case shown="True" w336 {
          tunnel: w333 -> [_ w358]
          tunnel: w329 -> [_ w365]
          tunnel: w332 -> [_ w361]
          tunnel: w335 -> [w352 w357]
          tunnel: [sgl[][] [] ("Data Array Out") w360] -> w327
          tunnel: [w352 w359] -> w334
          tunnel: w331 -> [_ w356]
          tunnel: w330 -> [_ w355]
          tunnel: [timestamp[] [] ("Multi Time Stamp") w354] -> w328
          frame #0 {
          }
          frame #1 {
            n153 = Quotient & Remainder(x=w361, y=w358) -> (floor(x/y)=w364:i32)  [unwired: 1 out]
            n154 = Initialize Array(sgl 0.0, w356, w364) -> (w363:sgl[][])
            n155 = call "SLL DE Decimate 2D Array.vi"("Multi Time Stamp"=w355, "Ref Array"=w363, "Decimation Rate"=w358, "Mod"=w357, "Data Array"=w365) -> ("Time array"=w354:timestamp[], "Mod Out"=w359:i32, "Data Array Out"=w360:sgl[][])  [unwired: 3 in, 1 out]
          }
        }
        n156 = Quotient & Remainder(x=w332, y=w340) -> (floor(x/y)=w325:i32)  [unwired: 1 out]
        n157 = Initialize Array(sgl 0.0, w331, w325) -> (w339:sgl[][])
        n158 = call "SLL DE Decimate 2D Array.vi"("Multi Time Stamp"=w330, "Ref Array"=w339, "Decimation Rate"=w340, "Mod"=w337, "Data Array"=w329) -> ("Mod Out"=w338:i32, "Data Array Out"=w326:sgl[][])  [unwired: 3 in, 2 out]
        n159 = Bundle By Name(cluster=w344, "Plot Details.Sample Value In"=w326, "Graph Mod"=w338, "Data Log To csv File"=w327, "File Mod"=w334, "Time Array"=w328) -> (w350:T4)
      }
      frame #6 {
        # "This case wil execute when Enable Record button is clicked.\nAll the Pre- Recording conditions are performed in this case after which \nrecording is done in \"Continue Recording\" Case. eg. opening the datalog\nfile and stuffs."
        n160 = Get Date/Time In Seconds() -> (seconds since 1Jan1904=w369:timestamp)
        n161 = Format Date/Time String(time format string (%c)="%m_%Y_%d_%H_%M_%S", seconds (now)=w369) -> (date/time string=w373:string)  [unwired: 1 in]
        n162 = Concatenate Strings("Log_" ("string"), w373, ".csv" ("string")) -> (w368:string)
        n163 = Build Path(base path="Data Save Folder Path", name or relative path=w368) -> (appended path=w366:path)
        n164 = Bundle By Name(cluster=w381, "Datalog Folder Path"=w366) -> (w380:T4)
        n165 = disable-structure shown="Disabled" {
          frame #0 {
            n166 = call "SLL DE File Looging Command LV2Global.vi"("Option"=SLL_DE_DO_Command_LV2Global_Options."Fire Event", "File Logging Option"=SLL_DE_File_Logging_Command_List."Start Logging") -> ()  [unwired: 1 in, 9 out]
          }
          frame #1 {
          }
        }
        n167 = call "SLL DE csv File Driver.vi"("Datalog Driver Cases"=SLL_DE_Virtual_Chart_Datalog_Driver_Options."Initialise", "error in(no error)"=w378, "Datalog path (use dialog)"=w366) -> ("error out"=w376:errorcluster)  [unwired: 4 in, 4 out]
        n168 = call "SLL DE csv File Driver.vi"("Datalog Driver Cases"=SLL_DE_Virtual_Chart_Datalog_Driver_Options."Write Headings", "error in(no error)"=w376) -> ("error out"=w375:errorcluster)  [unwired: 5 in, 4 out]
      }
      frame #7 {
        n169 = Unbundle By Name(w387) -> ("Time Array"=w384:timestamp[], "Data Log To csv File"=w385:sgl[][], "Record"=w388:bool, "Datalog Folder Path"=w389:path)
        n170 = case shown="True" w388 {
          tunnel: w390 -> [w392 w403]
          tunnel: [w392 w398] -> w386
          tunnel: w389 -> [_ w401]
          tunnel: w385 -> [_ w397]
          tunnel: w384 -> [_ w396]
          frame #0 {
          }
          frame #1 {
            # "Hold 70sec data in one file"
            n171 = call "SLL DE csv File Driver.vi"("Datalog Driver Cases"=SLL_DE_Virtual_Chart_Datalog_Driver_Options."Check File Size", "error in(no error)"=w403) -> ("error out"=w402:errorcluster, "size (in bytes)"=w395:i64)  [unwired: 5 in, 3 out]
            n172 = Greater?(x=w395, y=i64 15000000) -> (0:w393:bool)
            n173 = case shown="True" w393 {
              tunnel: w402 -> [w405 w410]
              tunnel: w401 -> [_ w409]
              tunnel: [w405 w406] -> w399
              frame #0 {
              }
              frame #1 {
                n174 = call "SLL DE csv File Driver.vi"("Datalog Driver Cases"=SLL_DE_Virtual_Chart_Datalog_Driver_Options."Initialise", "error in(no error)"=w410, "Datalog path (use dialog)"=w409) -> ("error out"=w407:errorcluster)  [unwired: 4 in, 4 out]
                n175 = call "SLL DE csv File Driver.vi"("Datalog Driver Cases"=SLL_DE_Virtual_Chart_Datalog_Driver_Options."Write Headings", "error in(no error)"=w407) -> ("error out"=w406:errorcluster)  [unwired: 5 in, 4 out]
              }
            }
            n176 = call "SLL DE csv File Driver.vi"("Datalog Driver Cases"=SLL_DE_Virtual_Chart_Datalog_Driver_Options."Write", "error in(no error)"=w399, "Data In"=w397, "Time Array"=w396) -> ("error out"=w398:errorcluster)  [unwired: 3 in, 4 out]
          }
        }
      }
      frame #8 {
        n177 = control-ref of="X-Scale"() -> (w412:refnum<vi>)
        n178 = Unbundle By Name(w413) -> ("Plot Details"=w416:T3)
        n179 = Build Array("Plot 1", "Plot 2", "Plot 3", "Plot 4") -> (w417:u16[])
        n180 = call "SLL DE Generate Plot LV2Global.vi"("Option"=SLL_DE_Get_Plot_LV2Global_Options."Get Plot", "error in (no error)"=w419, "X-Scale"=w412, "Plots"=w417, "Data Cluster"=w416) -> ("error IO"=w418:errorcluster)  [unwired: 5 in, 1 out]
      }
      frame #9 {
        # "Based on the configure plot details in both the axis, the \nramp detail for the particular channels corresponding to \nthe axis details will be plotted."
        n181 = case shown="True" "Hold Update" {
          tunnel: w427 -> [w429 w433]
          tunnel: [w429 w432] -> w426
          frame #0 {
          }
          frame #1 {
            n182 = call "SLL DE Generate Plot LV2Global.vi"("Option"=SLL_DE_Get_Plot_LV2Global_Options."Read Plot", "error in (no error)"=w433) -> ("error IO"=w432:errorcluster, "Plot data array"=→"Graph":T17)  [unwired: 8 in]
          }
        }
      }
      frame #10 {
        n183 = property on="Plot 1" class="Ring (strict)"() -> ("RingText.Text"=w444:string)  [unwired: 2 in, 2 out]
        n184 = property on="Plot 2" class="Ring (strict)"() -> ("RingText.Text"=w443:string)  [unwired: 2 in, 2 out]
        n185 = property on="Plot 3" class="Ring (strict)"() -> ("RingText.Text"=w442:string)  [unwired: 2 in, 2 out]
        n186 = property on="Plot 4" class="Ring (strict)"() -> ("RingText.Text"=w441:string)  [unwired: 2 in, 2 out]
        n187 = Unbundle By Name(w449) -> ("Plot Details.Plot 1"=w448:bool, "Plot Details.Plot 2"=w447:bool, "Plot Details.Plot 3"=w446:bool, "Plot Details.Plot 4"=w445:bool)
        n188 = Build Array(w448, w447, w446, w445) -> (w438:bool[])
        n189 = Build Array(w444, w443, w442, w441) -> (w435:string[])
        n190 = property on="Graph" class="XYGraph (strict)"() -> ("AnntList"=w436:T11)  [unwired: 2 in, 2 out]
        n191 = call "SLL Create Annotation List.vi"("Plot Name"=w435, "error in (no error)"=w434, "Plot Enable?"=w438, "Annotation Colour"=u32[] [16777215, 16728642, 982784, 16776704] ("Array"), "Annotation List"=w436) -> ("error out"=w440:errorcluster, "Annotation List Out"=w439:T11)  [unwired: 5 in]
        n192 = property on="Graph" class="XYGraph (strict)"("AnntList"=w439) -> ()  [unwired: 2 in, 2 out]
      }
      frame #11 {
        n193 = call "SLL DE File and folder info.vi"("error in (no error)"=w454) -> ("error out"=w451:errorcluster, "Report path"=w453:path)  [unwired: 5 in, 4 out]
        n194 = Get Date/Time In Seconds() -> (seconds since 1Jan1904=w456:timestamp)
        n195 = Format Date/Time String(time format string (%c)="%m_%Y_%d_%H_%M_%S", seconds (now)=w456) -> (date/time string=w460:string)  [unwired: 1 in]
        n196 = Concatenate Strings("Log_" ("string"), w460, ".bmp" ("string")) -> (w455:string)
        n197 = Build Path(base path=w453, name or relative path=w455) -> (appended path=w452:path)
        n198 = invoke on="Graph" class="XYGraph (strict)" method="Export Image Color"("File Type"=enum32{"BMP", "EPS", "EMF", "PICT"}."BMP", "Target"=enum32{"File", "Clipboard"}."File", "Path"=w452) -> ()  [unwired: 5 in, 8 out]
      }
      frame #12 {
        n199 = call "SLL DE Generate Plot LV2Global.vi"("Option"=SLL_DE_Get_Plot_LV2Global_Options."Init", "error in (no error)"=w475) -> ("error IO"=w474:errorcluster)  [unwired: 8 in, 1 out]
        n200 = Request Deallocation(TRUE ("flag")) -> ()
        n201 = local write "Graph"(T1 [] ("Graph")) -> ()
        n202 = property on="Graph" class="XYGraph (strict)"("AnntList"=T11 [] ("Annotation List")) -> ()  [unwired: 2 in, 2 out]
        n203 = Format Into String(format string="%s%s%s%s%s", SLL_DE_Virtual_Graph_Options."Get Values" ("SLL DE Virtual Chart Options"), SLL_DE_Virtual_Graph_Options."Config Plot" ("SLL DE Virtual Chart Options"), SLL_DE_Virtual_Graph_Options."Plot Ramp" ("SLL DE Virtual Chart Options"), SLL_DE_Virtual_Graph_Options."Datalog" ("SLL DE Virtual Chart Options"), SLL_DE_Virtual_Graph_Options."Add Plot Name" ("SLL DE Virtual Chart Options")) -> (resulting string=w465:string)  [unwired: 2 in, 1 out]
      }
      frame #13 {
        n204 = property on="Plot 1" class="Ring (strict)"() -> ("RingText.Text"=w493:string)  [unwired: 2 in, 2 out]
        n205 = property on="Plot 2" class="Ring (strict)"() -> ("RingText.Text"=w492:string)  [unwired: 2 in, 2 out]
        n206 = property on="Plot 3" class="Ring (strict)"() -> ("RingText.Text"=w491:string)  [unwired: 2 in, 2 out]
        n207 = property on="Plot 4" class="Ring (strict)"() -> ("RingText.Text"=w490:string)  [unwired: 2 in, 2 out]
        n208 = property on="X-Scale" class="Ring (strict)"() -> ("RingText.Text"=w489:string)  [unwired: 2 in, 2 out]
        n209 = local read "Y-Axis 2"() -> (w487:bool)
        n210 = local read "Y-Axis 1"() -> (w488:bool)
        n211 = Bundle By Name(cluster=T15 {"Plot 1"="", "Plot 2"="", "Plot 3"="", "Plot 4"="", "X Scale"="", "Y-Axis 2"=FALSE, "Y-Axis 1"=FALSE} ("Parameters"), "Plot 1"=w493, "Plot 2"=w492, "Plot 3"=w491, "Plot 4"=w490, "X Scale"=w489, "Y-Axis 2"=w487, "Y-Axis 1"=w488) -> (w483:T15)
        n212 = call "SLL DE Generate Plot LV2Global.vi"("Option"=SLL_DE_Get_Plot_LV2Global_Options."Read Plot", "error in (no error)"=w485) -> ("error IO"=w481:errorcluster, "Plot data array"=w482:T17)  [unwired: 8 in]
        n213 = call "SLL DE Print Chart.vi"("error in (no error)"=w481, "Plot data array"=w482, "Parameters"=w483) -> ("error out"=w480:errorcluster)  [unwired: 8 in]
      }
      frame #14 {
        n214 = call "SLL DE Three Button Error Dialog.vi"("Error In"=w500, "Window Title"="Error in Virtual Chart") -> ("Error Out"=w499:errorcluster, "Which Button?"=w502:T18)  [unwired: 8 in]
        n215 = case shown="\"Right Button\"" w502 {
          tunnel: ["Poll Events" ("Window Title") "Initialize" ("Window Title") "Exit" ("Window Title")] -> w497
          frame #0 {
          }
          frame #1 {
          }
          frame #2 {
          }
        }
        n216 = call <vilib>:"Clear Errors.vi"("error in (no error)"=w499) -> ("error out"=w496:errorcluster)  [unwired: 6 in]
      }
      frame #15 {
        n217 = call "SLL DE Generate Plot LV2Global.vi"("Option"=SLL_DE_Get_Plot_LV2Global_Options."Init", "error in (no error)"=w509) -> ("error IO"=w508:errorcluster)  [unwired: 8 in, 1 out]
        n218 = Request Deallocation(TRUE ("flag")) -> ()
        n219 = local write "Graph"(T1 [] ("Graph")) -> ()
        n220 = property on="Graph" class="XYGraph (strict)"("AnntList"=T11 [] ("Annotation List")) -> ()  [unwired: 2 in, 2 out]
      }
    }
  }
  n221 = Format Into String(format string="%s", SLL_DE_Virtual_Graph_Options."Error" ("SLL DE Virtual Chart Options")) -> ()  [unwired: 2 in, 2 out]
  n222 = property class="VI"(error in=w8, "Front Panel.Open"=TRUE ("Front Panel Window:Open")) -> (error out=→"error Out":errorcluster)  [unwired: 1 in, 1 out]
